vi "getSubtype.vi"(8 "error in (no error)":errorcluster, 11 "tBSONBinary in":refnum<class "tBSONBinary.lvclass">) -> (0 "error out":errorcluster, 2 "Type":T1 items=["Generic"=0, "Function"=1, "Binary (Old)"=2, "UUID"=3, "MD5"=5, "User Defined"=128], 3 "tBSONBinary out":refnum<class "tBSONBinary.lvclass">)   [LabVIEW 2013, in "BSON.lvlib" / "tBSONBinary.lvclass"]
uses:
  tBSONBinary.lvclass
  Subtype.ctl
  tBSONBinary.lvclass/tBSONBinary.ctl
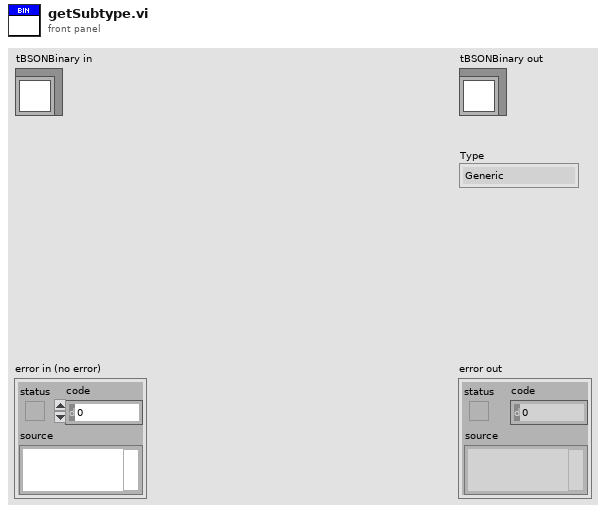
[diagram p1: front panel]
types:
  T1 = typedef "BSON.lvlib/tBSONBinary.lvclass/Subtype.ctl" = u8
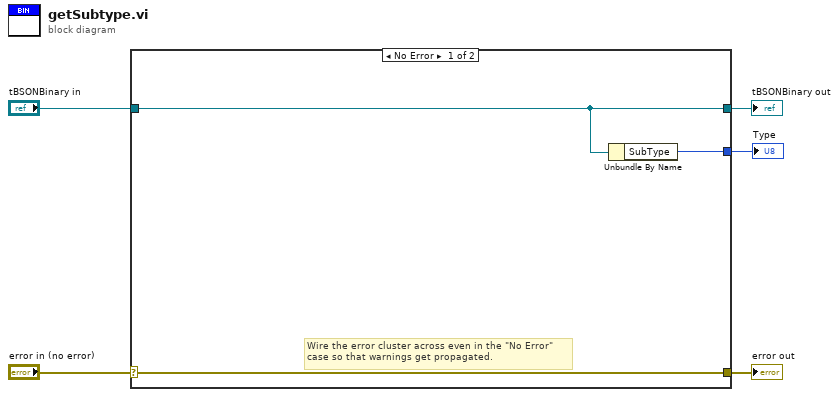
[diagram p0: block diagram]
diagram:
  n1 = case shown="No Error" "error in (no error)" {
    selector: "error in (no error)" -> [w8 w10]
    tunnel: [w8 w10] -> w4
    tunnel: [w7 w9] -> w2
    tunnel: "tBSONBinary in" -> [w7 w9]
    tunnel: [w6 _] -> w1
    frame No Error {
      # "Wire the error cluster across even in the \"No Error\"\ncase so that warnings get propagated."
      n2 = Unbundle By Name(w7) -> ("SubType"=w6:T1)
    }
    frame Error {
    }
  }
  "error out" <- w4
  "tBSONBinary out" <- w2
  "Type" <- w1
